vi "Main.vi"() -> ()   [LabVIEW 2011]
uses:
  Typedefs/Queue.ctl
  Typedefs/Queue cluster.ctl
  Typedefs/Cell details array.ctl
  Typedefs/Cell details cluster.ctl
  Typedefs/Scan settings.ctl
  Typedefs/StateEnum.ctl
panel:
  out "Server Status:":string
  out "Cell Settings Array 5":T1=[{"Measure?"=TRUE, "Area (cm^2)"=0.0, "Cell Label"="", "Cell Description"="", "Time between scans (s)"=0.0, "Cell Position"=1, "Scan settings in queue"=0, "Sample holder"=1.0, "User name"=""}, {"Measure?"=TRUE, "Area (cm^2)"=0.0, "Cell Label"="", "Cell Description"="", "Time between scans (s)"=0.0, "Cell Position"=2, "Scan settings in queue"=0, "Sample holder"=1.0, "User name"=""}, {"Measure?"=TRUE, "Area (cm^2)"=0.0, "Cell Label"="", "Cell Description"="", "Time between scans (s)"=0.0, "Cell Position"=3, "Scan settings in queue"=0, "Sample holder"=1.0, "User name"=""}, {"Measure?"=TRUE, "Area (cm^2)"=0.0, "Cell Label"="", "Cell Description"="", "Time between scans (s)"=0.0, "Cell Position"=4, "Scan settings in queue"=0, "Sample holder"=1.0, "User name"=""}, {"Measure?"=TRUE, "Area (cm^2)"=0.0, "Cell Label"="", "Cell Description"="", "Time between scans (s)"=0.0, "Cell Position"=5, "Scan settings in queue"=0, "Sample holder"=1.0, "User name"=""}, {"Measure?"=TRUE, "Area (cm^2)"=0.0, "Cell Label"="", "Cell Description"="", "Time between scans (s)"=0.0, "Cell Position"=6, "Scan settings in queue"=0, "Sample holder"=1.0, "User name"=""}, {"Measure?"=TRUE, "Area (cm^2)"=0.0, "Cell Label"="", "Cell Description"="", "Time between scans (s)"=0.0, "Cell Position"=7, "Scan settings in queue"=0, "Sample holder"=1.0, "User name"=""}, {"Measure?"=TRUE, "Area (cm^2)"=0.0, "Cell Label"="", "Cell Description"="", "Time between scans (s)"=0.0, "Cell Position"=8, "Scan settings in queue"=0, "Sample holder"=1.0, "User name"=""}, {"Measure?"=TRUE, "Area (cm^2)"=0.0, "Cell Label"="", "Cell Description"="", "Time between scans (s)"=0.0, "Cell Position"=9, "Scan settings in queue"=0, "Sample holder"=1.0, "User name"=""}, {"Measure?"=TRUE, "Area (cm^2)"=0.0, "Cell Label"="", "Cell Description"="", "Time between scans (s)"=0.0, "Cell Position"=10, "Scan settings in queue"=0, "Sample holder"=1.0, "User name"=""}, {"Measure?"=TRUE, "Area (cm^2)"=0.0, "Cell Label"="", "Cell Description"="", "Time between scans (s)"=0.0, "Cell Position"=11, "Scan settings in queue"=0, "Sample holder"=1.0, "User name"=""}, {"Measure?"=TRUE, "Area (cm^2)"=0.0, "Cell Label"="", "Cell Description"="", "Time between scans (s)"=0.0, "Cell Position"=12, "Scan settings in queue"=0, "Sample holder"=1.0, "User name"=""}, {"Measure?"=TRUE, "Area (cm^2)"=0.0, "Cell Label"="", "Cell Description"="", "Time between scans (s)"=0.0, "Cell Position"=13, "Scan settings in queue"=0, "Sample holder"=1.0, "User name"=""}, {"Measure?"=TRUE, "Area (cm^2)"=0.0, "Cell Label"="", "Cell Description"="", "Time between scans (s)"=0.0, "Cell Position"=14, "Scan settings in queue"=0, "Sample holder"=1.0, "User name"=""}, {"Measure?"=TRUE, "Area (cm^2)"=0.0, "Cell Label"="", "Cell Description"="", "Time between scans (s)"=0.0, "Cell Position"=15, "Scan settings in queue"=0, "Sample holder"=1.0, "User name"=""}, {"Measure?"=TRUE, "Area (cm^2)"=0.0, "Cell Label"="", "Cell Description"="", "Time between scans (s)"=0.0, "Cell Position"=16, "Scan settings in queue"=0, "Sample holder"=1.0, "User name"=""}] {"Scan settings in queue" items=["Standard"]}
  in  "Tab Control":T3(tab)
  in  "Cell Settings Array 1":T1=[{"Measure?"=TRUE, "Area (cm^2)"=0.0, "Cell Label"="", "Cell Description"="", "Time between scans (s)"=0.0, "Cell Position"=1, "Scan settings in queue"=0, "Sample holder"=1.0, "User name"=""}, {"Measure?"=TRUE, "Area (cm^2)"=0.0, "Cell Label"="", "Cell Description"="", "Time between scans (s)"=0.0, "Cell Position"=2, "Scan settings in queue"=0, "Sample holder"=1.0, "User name"=""}, {"Measure?"=TRUE, "Area (cm^2)"=0.0, "Cell Label"="", "Cell Description"="", "Time between scans (s)"=0.0, "Cell Position"=3, "Scan settings in queue"=0, "Sample holder"=1.0, "User name"=""}, {"Measure?"=TRUE, "Area (cm^2)"=0.0, "Cell Label"="", "Cell Description"="", "Time between scans (s)"=0.0, "Cell Position"=4, "Scan settings in queue"=0, "Sample holder"=1.0, "User name"=""}, {"Measure?"=TRUE, "Area (cm^2)"=0.0, "Cell Label"="", "Cell Description"="", "Time between scans (s)"=0.0, "Cell Position"=5, "Scan settings in queue"=0, "Sample holder"=1.0, "User name"=""}, {"Measure?"=TRUE, "Area (cm^2)"=0.0, "Cell Label"="", "Cell Description"="", "Time between scans (s)"=0.0, "Cell Position"=6, "Scan settings in queue"=0, "Sample holder"=1.0, "User name"=""}, {"Measure?"=TRUE, "Area (cm^2)"=0.0, "Cell Label"="", "Cell Description"="", "Time between scans (s)"=0.0, "Cell Position"=7, "Scan settings in queue"=0, "Sample holder"=1.0, "User name"=""}, {"Measure?"=TRUE, "Area (cm^2)"=0.0, "Cell Label"="", "Cell Description"="", "Time between scans (s)"=0.0, "Cell Position"=8, "Scan settings in queue"=0, "Sample holder"=1.0, "User name"=""}, {"Measure?"=TRUE, "Area (cm^2)"=0.0, "Cell Label"="", "Cell Description"="", "Time between scans (s)"=0.0, "Cell Position"=9, "Scan settings in queue"=0, "Sample holder"=1.0, "User name"=""}, {"Measure?"=TRUE, "Area (cm^2)"=0.0, "Cell Label"="", "Cell Description"="", "Time between scans (s)"=0.0, "Cell Position"=10, "Scan settings in queue"=0, "Sample holder"=1.0, "User name"=""}, {"Measure?"=TRUE, "Area (cm^2)"=0.0, "Cell Label"="", "Cell Description"="", "Time between scans (s)"=0.0, "Cell Position"=11, "Scan settings in queue"=0, "Sample holder"=1.0, "User name"=""}, {"Measure?"=TRUE, "Area (cm^2)"=0.0, "Cell Label"="", "Cell Description"="", "Time between scans (s)"=0.0, "Cell Position"=12, "Scan settings in queue"=0, "Sample holder"=1.0, "User name"=""}, {"Measure?"=TRUE, "Area (cm^2)"=0.0, "Cell Label"="", "Cell Description"="", "Time between scans (s)"=0.0, "Cell Position"=13, "Scan settings in queue"=0, "Sample holder"=1.0, "User name"=""}, {"Measure?"=TRUE, "Area (cm^2)"=0.0, "Cell Label"="", "Cell Description"="", "Time between scans (s)"=0.0, "Cell Position"=14, "Scan settings in queue"=0, "Sample holder"=1.0, "User name"=""}, {"Measure?"=TRUE, "Area (cm^2)"=0.0, "Cell Label"="", "Cell Description"="", "Time between scans (s)"=0.0, "Cell Position"=15, "Scan settings in queue"=0, "Sample holder"=1.0, "User name"=""}, {"Measure?"=TRUE, "Area (cm^2)"=0.0, "Cell Label"="", "Cell Description"="", "Time between scans (s)"=0.0, "Cell Position"=16, "Scan settings in queue"=0, "Sample holder"=1.0, "User name"=""}] {"Scan settings in queue" items=["David_Std", "Inverted", "Standard"]}
  in  "Upload from Spreadsheet?":bool
  in  "Upload Spreadsheet path":path=path "C:/Solar_Cell_Stability/Cell Details/Sample holder A.txt"
  in  "Save to Spreadsheet?":bool
  in  "Save Spreadsheet Path":path=path "C:/Solar_Cell_Stability/Cell Details/Sample holder A.txt"
  in  "Cell Settings Array 2":T1=[{"Measure?"=TRUE, "Area (cm^2)"=0.0, "Cell Label"="", "Cell Description"="", "Time between scans (s)"=0.0, "Cell Position"=1, "Scan settings in queue"=0, "Sample holder"=2.0, "User name"=""}, {"Measure?"=TRUE, "Area (cm^2)"=0.0, "Cell Label"="", "Cell Description"="", "Time between scans (s)"=0.0, "Cell Position"=2, "Scan settings in queue"=0, "Sample holder"=2.0, "User name"=""}, {"Measure?"=TRUE, "Area (cm^2)"=0.0, "Cell Label"="", "Cell Description"="", "Time between scans (s)"=0.0, "Cell Position"=3, "Scan settings in queue"=0, "Sample holder"=2.0, "User name"=""}, {"Measure?"=TRUE, "Area (cm^2)"=0.0, "Cell Label"="", "Cell Description"="", "Time between scans (s)"=0.0, "Cell Position"=4, "Scan settings in queue"=0, "Sample holder"=2.0, "User name"=""}, {"Measure?"=TRUE, "Area (cm^2)"=0.0, "Cell Label"="", "Cell Description"="", "Time between scans (s)"=0.0, "Cell Position"=5, "Scan settings in queue"=0, "Sample holder"=2.0, "User name"=""}, {"Measure?"=TRUE, "Area (cm^2)"=0.0, "Cell Label"="", "Cell Description"="", "Time between scans (s)"=0.0, "Cell Position"=6, "Scan settings in queue"=0, "Sample holder"=2.0, "User name"=""}, {"Measure?"=TRUE, "Area (cm^2)"=0.0, "Cell Label"="", "Cell Description"="", "Time between scans (s)"=0.0, "Cell Position"=7, "Scan settings in queue"=0, "Sample holder"=2.0, "User name"=""}, {"Measure?"=TRUE, "Area (cm^2)"=0.0, "Cell Label"="", "Cell Description"="", "Time between scans (s)"=0.0, "Cell Position"=8, "Scan settings in queue"=0, "Sample holder"=2.0, "User name"=""}, {"Measure?"=TRUE, "Area (cm^2)"=0.0, "Cell Label"="", "Cell Description"="", "Time between scans (s)"=0.0, "Cell Position"=9, "Scan settings in queue"=0, "Sample holder"=2.0, "User name"=""}, {"Measure?"=TRUE, "Area (cm^2)"=0.0, "Cell Label"="", "Cell Description"="", "Time between scans (s)"=0.0, "Cell Position"=10, "Scan settings in queue"=0, "Sample holder"=2.0, "User name"=""}, {"Measure?"=TRUE, "Area (cm^2)"=0.0, "Cell Label"="", "Cell Description"="", "Time between scans (s)"=0.0, "Cell Position"=11, "Scan settings in queue"=0, "Sample holder"=2.0, "User name"=""}, {"Measure?"=TRUE, "Area (cm^2)"=0.0, "Cell Label"="", "Cell Description"="", "Time between scans (s)"=0.0, "Cell Position"=12, "Scan settings in queue"=0, "Sample holder"=2.0, "User name"=""}, {"Measure?"=TRUE, "Area (cm^2)"=0.0, "Cell Label"="", "Cell Description"="", "Time between scans (s)"=0.0, "Cell Position"=13, "Scan settings in queue"=0, "Sample holder"=2.0, "User name"=""}, {"Measure?"=TRUE, "Area (cm^2)"=0.0, "Cell Label"="", "Cell Description"="", "Time between scans (s)"=0.0, "Cell Position"=14, "Scan settings in queue"=0, "Sample holder"=2.0, "User name"=""}, {"Measure?"=TRUE, "Area (cm^2)"=0.0, "Cell Label"="", "Cell Description"="", "Time between scans (s)"=0.0, "Cell Position"=15, "Scan settings in queue"=0, "Sample holder"=2.0, "User name"=""}, {"Measure?"=TRUE, "Area (cm^2)"=0.0, "Cell Label"="", "Cell Description"="", "Time between scans (s)"=0.0, "Cell Position"=16, "Scan settings in queue"=0, "Sample holder"=2.0, "User name"=""}] {"Scan settings in queue" items=["David_Std", "Inverted", "Standard"]}
  in  "Upload Spreadsheet path 2":path=path "C:/Solar_Cell_Stability/Cell Details/Sample holder B.txt"
  in  "Upload from Spreadsheet? 2":bool
  in  "Save Spreadsheet Path 2":path=path "C:/Solar_Cell_Stability/Cell Details/Sample holder B.txt"
  in  "Save to Spreadsheet?  2":bool
  in  "Cell Settings Array 3":T1=[{"Measure?"=TRUE, "Area (cm^2)"=0.0, "Cell Label"="", "Cell Description"="", "Time between scans (s)"=0.0, "Cell Position"=1, "Scan settings in queue"=0, "Sample holder"=3.0, "User name"=""}, {"Measure?"=TRUE, "Area (cm^2)"=0.0, "Cell Label"="", "Cell Description"="", "Time between scans (s)"=0.0, "Cell Position"=2, "Scan settings in queue"=0, "Sample holder"=3.0, "User name"=""}, {"Measure?"=TRUE, "Area (cm^2)"=0.0, "Cell Label"="", "Cell Description"="", "Time between scans (s)"=0.0, "Cell Position"=3, "Scan settings in queue"=0, "Sample holder"=3.0, "User name"=""}, {"Measure?"=TRUE, "Area (cm^2)"=0.0, "Cell Label"="", "Cell Description"="", "Time between scans (s)"=0.0, "Cell Position"=4, "Scan settings in queue"=0, "Sample holder"=3.0, "User name"=""}, {"Measure?"=TRUE, "Area (cm^2)"=0.0, "Cell Label"="", "Cell Description"="", "Time between scans (s)"=0.0, "Cell Position"=5, "Scan settings in queue"=0, "Sample holder"=3.0, "User name"=""}, {"Measure?"=TRUE, "Area (cm^2)"=0.0, "Cell Label"="", "Cell Description"="", "Time between scans (s)"=0.0, "Cell Position"=6, "Scan settings in queue"=0, "Sample holder"=3.0, "User name"=""}, {"Measure?"=TRUE, "Area (cm^2)"=0.0, "Cell Label"="", "Cell Description"="", "Time between scans (s)"=0.0, "Cell Position"=7, "Scan settings in queue"=0, "Sample holder"=3.0, "User name"=""}, {"Measure?"=TRUE, "Area (cm^2)"=0.0, "Cell Label"="", "Cell Description"="", "Time between scans (s)"=0.0, "Cell Position"=8, "Scan settings in queue"=0, "Sample holder"=3.0, "User name"=""}, {"Measure?"=TRUE, "Area (cm^2)"=0.0, "Cell Label"="", "Cell Description"="", "Time between scans (s)"=0.0, "Cell Position"=9, "Scan settings in queue"=0, "Sample holder"=3.0, "User name"=""}, {"Measure?"=TRUE, "Area (cm^2)"=0.0, "Cell Label"="", "Cell Description"="", "Time between scans (s)"=0.0, "Cell Position"=10, "Scan settings in queue"=0, "Sample holder"=3.0, "User name"=""}, {"Measure?"=TRUE, "Area (cm^2)"=0.0, "Cell Label"="", "Cell Description"="", "Time between scans (s)"=0.0, "Cell Position"=11, "Scan settings in queue"=0, "Sample holder"=3.0, "User name"=""}, {"Measure?"=TRUE, "Area (cm^2)"=0.0, "Cell Label"="", "Cell Description"="", "Time between scans (s)"=0.0, "Cell Position"=12, "Scan settings in queue"=0, "Sample holder"=3.0, "User name"=""}, {"Measure?"=TRUE, "Area (cm^2)"=0.0, "Cell Label"="", "Cell Description"="", "Time between scans (s)"=0.0, "Cell Position"=13, "Scan settings in queue"=0, "Sample holder"=3.0, "User name"=""}, {"Measure?"=TRUE, "Area (cm^2)"=0.0, "Cell Label"="", "Cell Description"="", "Time between scans (s)"=0.0, "Cell Position"=14, "Scan settings in queue"=0, "Sample holder"=3.0, "User name"=""}, {"Measure?"=TRUE, "Area (cm^2)"=0.0, "Cell Label"="", "Cell Description"="", "Time between scans (s)"=0.0, "Cell Position"=15, "Scan settings in queue"=0, "Sample holder"=3.0, "User name"=""}, {"Measure?"=TRUE, "Area (cm^2)"=0.0, "Cell Label"="", "Cell Description"="", "Time between scans (s)"=0.0, "Cell Position"=16, "Scan settings in queue"=0, "Sample holder"=3.0, "User name"=""}] {"Scan settings in queue" items=["David_Std", "Inverted", "Standard"]}
  in  "Upload Spreadsheet path 3":path=path "C:/Solar_Cell_Stability/Cell Details/Sample holder C.txt"
  in  "Upload from Spreadsheet? 3":bool
  in  "Save Spreadsheet Path 3":path=path "C:/Solar_Cell_Stability/Cell Details/Sample holder C.txt"
  in  "Save to Spreadsheet?  3":bool
  in  "Cell Settings Array 4":T1=[{"Measure?"=TRUE, "Area (cm^2)"=0.0, "Cell Label"="", "Cell Description"="", "Time between scans (s)"=0.0, "Cell Position"=1, "Scan settings in queue"=0, "Sample holder"=4.0, "User name"=""}, {"Measure?"=TRUE, "Area (cm^2)"=0.0, "Cell Label"="", "Cell Description"="", "Time between scans (s)"=0.0, "Cell Position"=2, "Scan settings in queue"=0, "Sample holder"=4.0, "User name"=""}, {"Measure?"=TRUE, "Area (cm^2)"=0.0, "Cell Label"="", "Cell Description"="", "Time between scans (s)"=0.0, "Cell Position"=3, "Scan settings in queue"=0, "Sample holder"=4.0, "User name"=""}, {"Measure?"=TRUE, "Area (cm^2)"=0.0, "Cell Label"="", "Cell Description"="", "Time between scans (s)"=0.0, "Cell Position"=4, "Scan settings in queue"=0, "Sample holder"=4.0, "User name"=""}, {"Measure?"=TRUE, "Area (cm^2)"=0.0, "Cell Label"="", "Cell Description"="", "Time between scans (s)"=0.0, "Cell Position"=5, "Scan settings in queue"=0, "Sample holder"=4.0, "User name"=""}, {"Measure?"=TRUE, "Area (cm^2)"=0.0, "Cell Label"="", "Cell Description"="", "Time between scans (s)"=0.0, "Cell Position"=6, "Scan settings in queue"=0, "Sample holder"=4.0, "User name"=""}, {"Measure?"=TRUE, "Area (cm^2)"=0.0, "Cell Label"="", "Cell Description"="", "Time between scans (s)"=0.0, "Cell Position"=7, "Scan settings in queue"=0, "Sample holder"=4.0, "User name"=""}, {"Measure?"=TRUE, "Area (cm^2)"=0.0, "Cell Label"="", "Cell Description"="", "Time between scans (s)"=0.0, "Cell Position"=8, "Scan settings in queue"=0, "Sample holder"=4.0, "User name"=""}, {"Measure?"=TRUE, "Area (cm^2)"=0.0, "Cell Label"="", "Cell Description"="", "Time between scans (s)"=0.0, "Cell Position"=9, "Scan settings in queue"=0, "Sample holder"=4.0, "User name"=""}, {"Measure?"=TRUE, "Area (cm^2)"=0.0, "Cell Label"="", "Cell Description"="", "Time between scans (s)"=0.0, "Cell Position"=10, "Scan settings in queue"=0, "Sample holder"=4.0, "User name"=""}, {"Measure?"=TRUE, "Area (cm^2)"=0.0, "Cell Label"="", "Cell Description"="", "Time between scans (s)"=0.0, "Cell Position"=11, "Scan settings in queue"=0, "Sample holder"=4.0, "User name"=""}, {"Measure?"=TRUE, "Area (cm^2)"=0.0, "Cell Label"="", "Cell Description"="", "Time between scans (s)"=0.0, "Cell Position"=12, "Scan settings in queue"=0, "Sample holder"=4.0, "User name"=""}, {"Measure?"=TRUE, "Area (cm^2)"=0.0, "Cell Label"="", "Cell Description"="", "Time between scans (s)"=0.0, "Cell Position"=13, "Scan settings in queue"=0, "Sample holder"=4.0, "User name"=""}, {"Measure?"=TRUE, "Area (cm^2)"=0.0, "Cell Label"="", "Cell Description"="", "Time between scans (s)"=0.0, "Cell Position"=14, "Scan settings in queue"=0, "Sample holder"=4.0, "User name"=""}, {"Measure?"=TRUE, "Area (cm^2)"=0.0, "Cell Label"="", "Cell Description"="", "Time between scans (s)"=0.0, "Cell Position"=15, "Scan settings in queue"=0, "Sample holder"=4.0, "User name"=""}, {"Measure?"=TRUE, "Area (cm^2)"=0.0, "Cell Label"="", "Cell Description"="", "Time between scans (s)"=0.0, "Cell Position"=16, "Scan settings in queue"=0, "Sample holder"=4.0, "User name"=""}] {"Scan settings in queue" items=["David_Std", "Inverted", "Standard"]}
  in  "Upload Spreadsheet path 4":path=path "C:/Solar_Cell_Stability/Cell Details/Sample holder D.txt"
  in  "Upload from Spreadsheet? 4":bool
  in  "Save Spreadsheet Path 4":path=path "C:/Solar_Cell_Stability/Cell Details/Sample holder D.txt"
  in  "Save to Spreadsheet?  4":bool
  in  "Stop Scan":bool
  in  "Start Scan":bool
  out "Table":string[][](table)
  in  "Upload to the Queue":bool
  in  "Stop Scan 2":bool
  out "J-V Curve":cluster{"Y":dbl[], "Y":dbl[]}[](graph)
  out "Max. Power Stabilization":cluster{"Y":dbl[], "Y":dbl[]}[](graph)
  in  "Scan Settings JV":T4={"Light intensity (Suns)"=1.0, "Pre-bias time (s)"=5.0, "Maximum voltage (V)"=0.0, "Minimum voltage (V)"=-1.4, "Range Options"=0, "1st scan FB to SC?"=TRUE, "Step Size (V)"=0.01, "Source Delay (s)"=0.01, "Inverted device"=FALSE, "Measure stabilized power output"=TRUE, "Stabilzation time (s)"=40.0, "Use Vmp from JV scan"=TRUE, "Stabization voltage (V)"=0.8, "Only stabilize best pixels"=TRUE, "Number of pixels to stabilize \nper substrate"=0, "Stabilization time step (s)"=1.0, "Use max power tracking"=FALSE, "Pre-bias voltage (V)"=-1.4, "No. of data point averages"=1.0, "No. of J-V averages"=1.0, "Integration time (ms)"=200.0} {"Integration time (ms)" min=0.2 max=200.0; "Number of pixels to stabilize \nper substrate" items=["1", "2", "3", "4", "5", "6", "7", "8"]; "Range Options" items=["Auto Range", "100 uA", "1 mA", "10 mA", "100 mA", "1A"]}
  in  "Save new settings as...":string
  in  "Save new settings":bool
  in  "Show saved settings":u16(ring) items=["David_Std", "Inverted", "Standard"]
  in  "Queue":T5 {"Scan settings in queue" items=["David_Std", "Inverted", "Standard"]; "Time of the last scan (s)" format="%<%H:%M:%S>t"; "When did you stick it in?" format="%<%H:%M:%S>t"; "Time to next scan (s)" format="%<%H:%M:%S>t"; "Time in rig (s)" format="%<%H:%M:%S>t"}
  out "TIMER":dbl format="%<%H:%M:%S>t"
  # "Cell Ageing"
  # "Time between Scans (s)"
  # "Area\n(cm^2)"
  # "Cell\nPosition"
  # "Sample\nHolder"
  # "On = working\nOff = not working"
  # "Label"
  # "User Name"
  # "Comment"
  # "Scan Settings"
  # "Time between Scans (s)"
  # "Area\n(cm^2)"
  # "Cell\nPosition"
  # "Sample\nHolder"
  # "On = working\nOff = not working"
  # "Label"
  # "User Name"
  # "Comment"
  # "Scan Settings"
  # "Time between Scans (s)"
  # "Area\n(cm^2)"
  # "Cell\nPosition"
  # "Sample\nHolder"
  # "On = working\nOff = not working"
  # "Label"
  # "User Name"
  # "Comment"
  # "Scan Settings"
  # "Time between Scans (s)"
  # "Area\n(cm^2)"
  # "Cell\nPosition"
  # "Sample\nHolder"
  # "On = working\nOff = not working"
  # "Label"
  # "User Name"
  # "Comment"
  # "Scan Settings"
  # "Time\n(s)"
  # "Light\nintensity"
  # "Cell\nLabel"
  # "Pixel\nNo."
  # "Scan\nNo."
  # "File\nPath"
  # "Area"
  # "Jsc"
  # "Voc"
  # "PCE"
  # "FF"
  # "Vmp"
  # "Comment"
  # "N.B. Voltage is applied to TCO electrode,\ni.e. the power generating quadrant is at \nnegative voltage for standard devices but \nat positive voltage for inverted devices."
  # "Area\n(cm^2)"
  # "Scan\nwait (s)"
  # "Cell \nposition"
  # "Time in rig\n(hrs)"
  # "Time to next scan (hrs)"
  # "Scan\nnumber"
  # "Time\nZero"
  # "Time of \nlast scan"
  # "Sample\nHolder"
  # "On = working\nOff = not working"
  # "Label"
  # "User"
  # "Comment"
  # "Scan Settings"
  # "WARNING: Deviating from these instructions may have serious consequences including massive data loss!\n\n\nBASIC OPERATION:\n\nFill out the cell details for each cell in each sample holder on the \"Sample Holder #\" tabs. For easy data analysis later, add an experiment indicator to\nthe \"Comments\" field. Be sure to complete all the information for each cell. If any boxes are blank, that cell won't be measured.\n\nGo to the \"Start/Stop Scan\" tab. Click the \"Initialise/Refresh Queue\" button. Check the \"Queue\" tab to make sure the the cell details have been added.\n\nOn the \"Start/Stop Scan\" tab click the \"Start Scan\" button. The cells in the queue will start to be measured.\n\n\n\nTO ADD CUSTOM SCAN SETTINGS:\n\nGo to the \"Scan Settings\" tab.\n\nInsert a new name into the \"Scan Setting Name\" box. Fill out the details in the pane and then press \"Save\". Your new settings are now accessible to\nselect when filling in the sample details in the \"Sample Holder #\" tabs.\n\nExisting settings can be viewed by selecting the appropriate option from the \"Show Scan Settings\" dropdown box.\n\n\n\nTO ADD/REMOVE/SWAP CELLS AND CONTINUE MEASUREMENT:\n\nGo to the \"Start/Stop Scan\" tab. Click the \"Stop Scan\" button. Wait for all the pixels on the current quad to finish measuring.\n\nAdd/change the required cells and repeat \"Basic Operation\".\n\n\n\nADDITIONAL INFORMATION\n\nDuring the measurement, only the \"Stop Scan\" button is functional. No changes can be made whilst measurements are running. Any attempts to \npress other buttons during measurements will result in a program crash.\n\nYou cannot update the comments box once a cell has been uploaded to the queue."
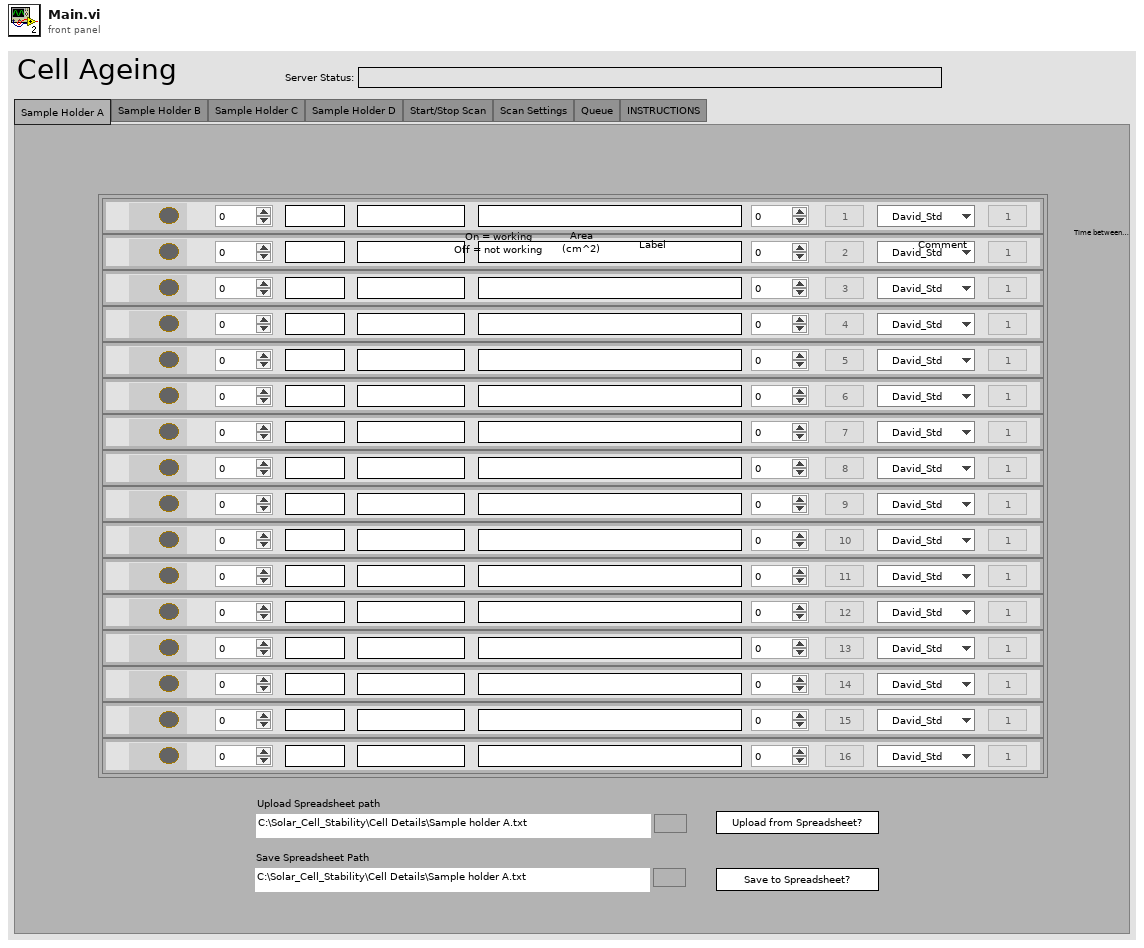
[diagram p1: front panel]
types:
  T1 = typedef "Cell details array.ctl" = T2[]
  T2 = typedef "Cell details cluster.ctl" = cluster{"Measure?":bool, "Area (cm^2)":dbl, "Cell Label":string, "Cell Description":string, "Time between scans (s)":dbl, "Cell Position":i32, "Scan settings in queue":u16, "Sample holder":dbl, "User name":string}
  T3 = enum32{"Sample Holder A", "Sample Holder B", "Sample Holder C", "Sample Holder D", "Start/Stop Scan", "Scan Settings", "Queue", "INSTRUCTIONS"}
  T4 = typedef "Scan settings.ctl" = cluster{"Light intensity (Suns)":dbl, "Pre-bias time (s)":dbl, "Maximum voltage (V)":dbl, "Minimum voltage (V)":dbl, "Range Options":u16, "1st scan FB to SC?":bool, "Step Size (V)":dbl, "Source Delay (s)":dbl, "Inverted device":bool, "Measure stabilized power output":bool, "Stabilzation time (s)":dbl, "Use Vmp from JV scan":bool, "Stabization voltage (V)":dbl, "Only stabilize best pixels":bool, "Number of pixels to stabilize \nper substrate":u16, "Stabilization time step (s)":dbl, "Use max power tracking":bool, "Pre-bias voltage (V)":dbl, "No. of data point averages":dbl, "No. of J-V averages":dbl, "Integration time (ms)":dbl}
  T5 = typedef "Queue.ctl" = T6[]
  T6 = typedef "Queue cluster.ctl" = cluster{"Measure?":bool, "Area (cm^2)":dbl, "Cell Label":string, "Cell Description":string, "Cell Position":i32, "Time in rig (s)":dbl, "Time to next scan (s)":dbl, "Scan number":dbl, "When did you stick it in?":dbl, "Time between scans (s)":dbl, "Time of the last scan (s)":dbl, "Scan settings in queue":u16, "Sample Holder":dbl, "User Name":string}
  T7 = typedef "StateEnum.ctl" = enum16{"Idle", "Measure"}
  T8 = enum8{"Enabled", "Disabled", "Disabled and Grayed Out"}
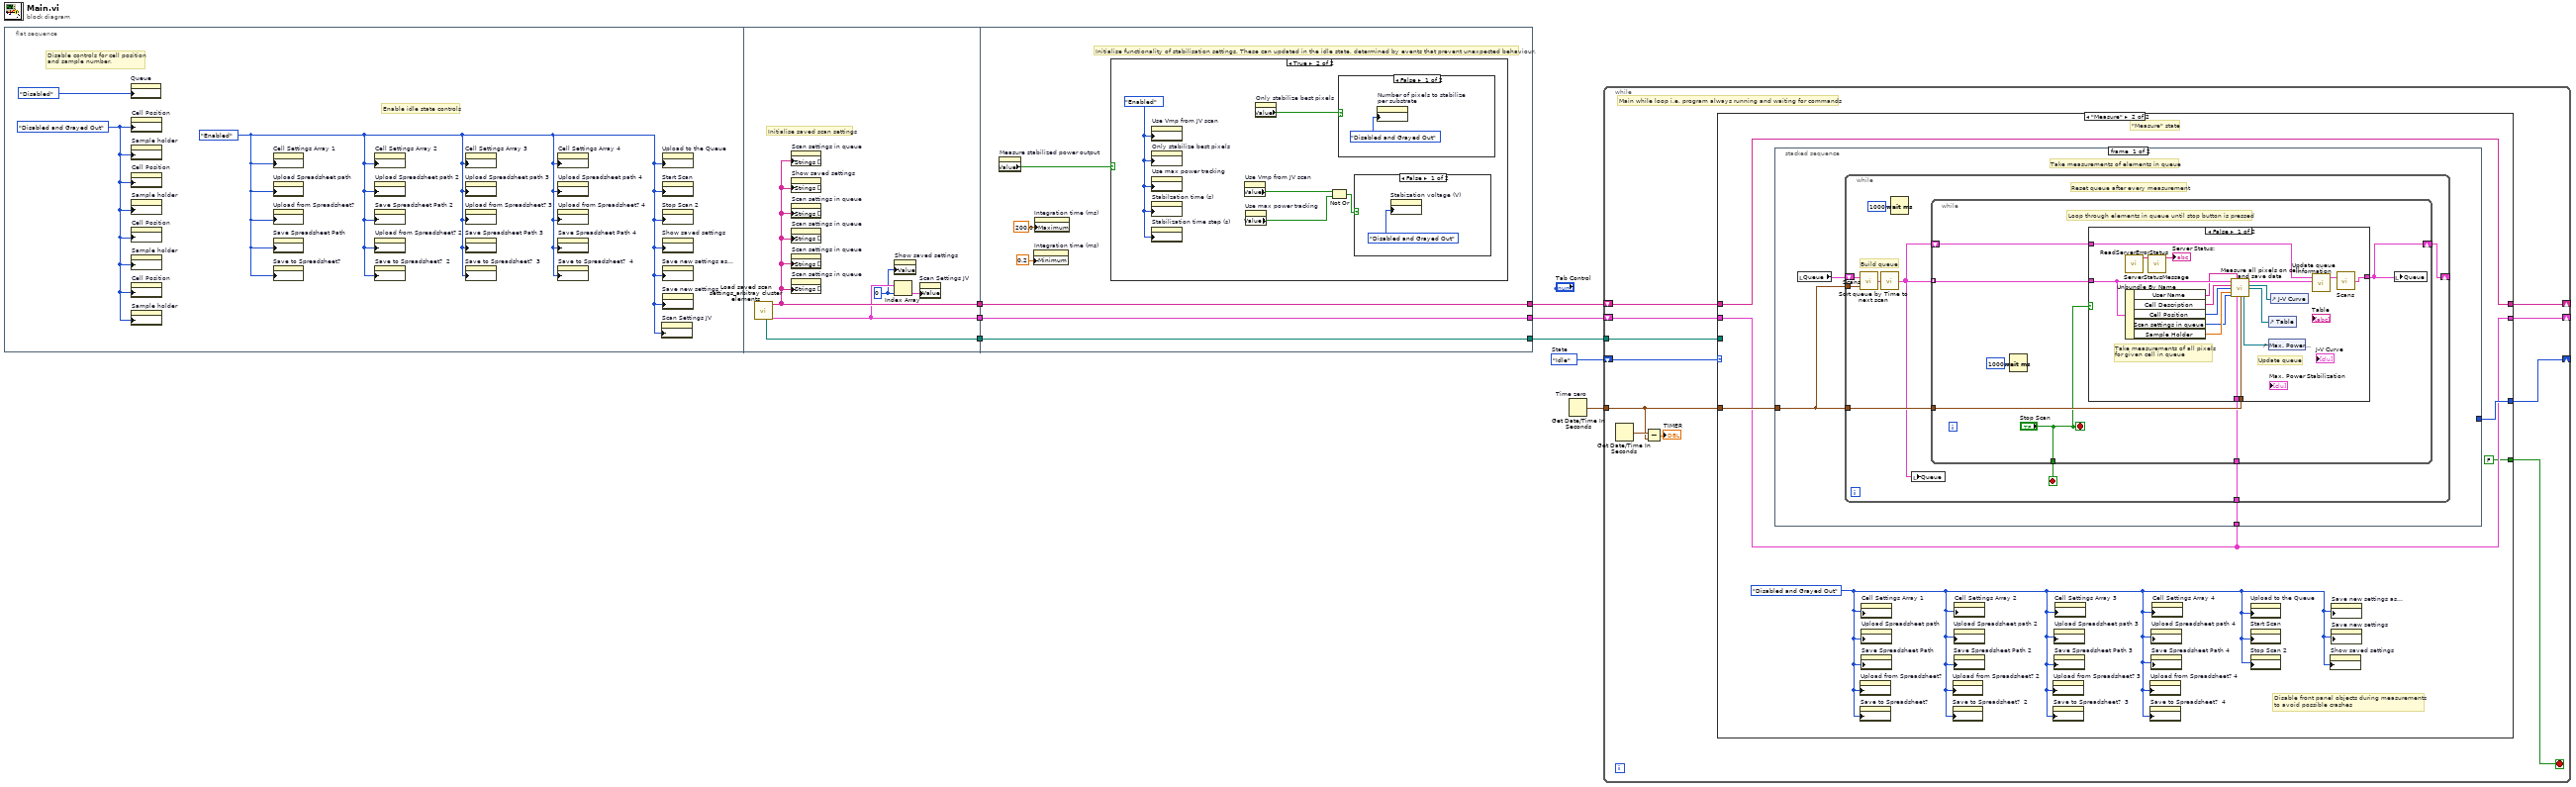
[diagram p0: block diagram]
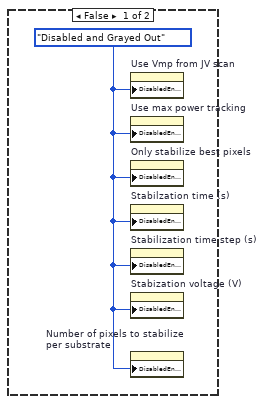
[diagram p2: hidden frame]
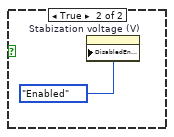
[diagram p3: hidden frame]
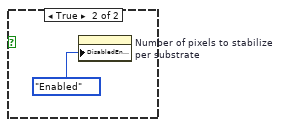
[diagram p4: hidden frame]
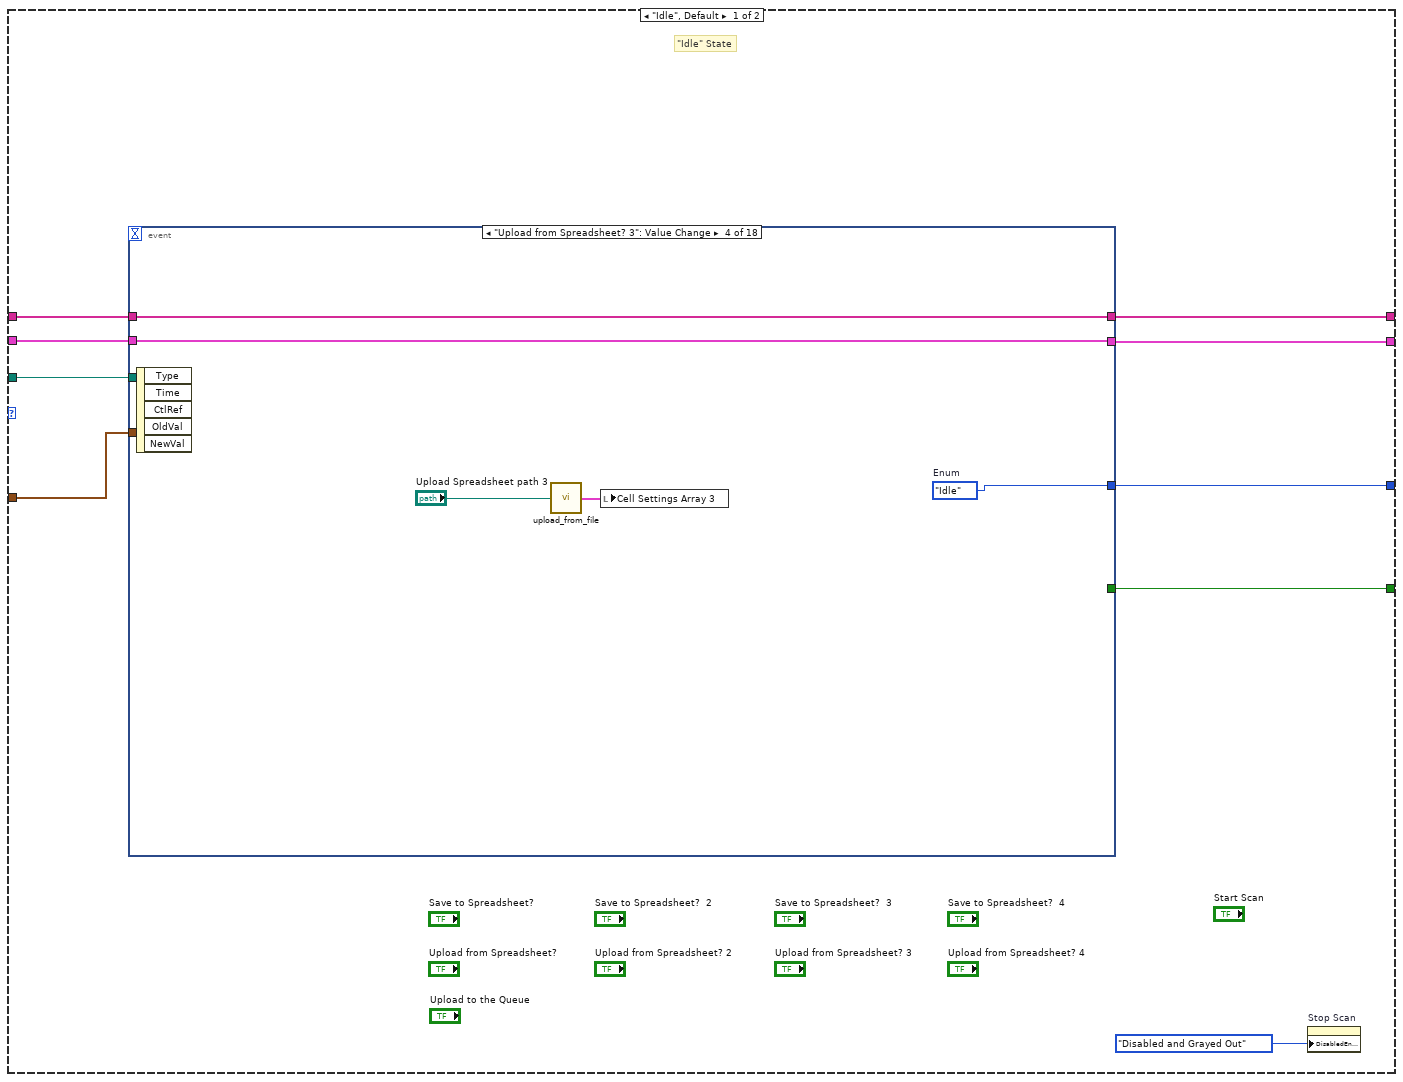
[diagram p5: hidden frame]
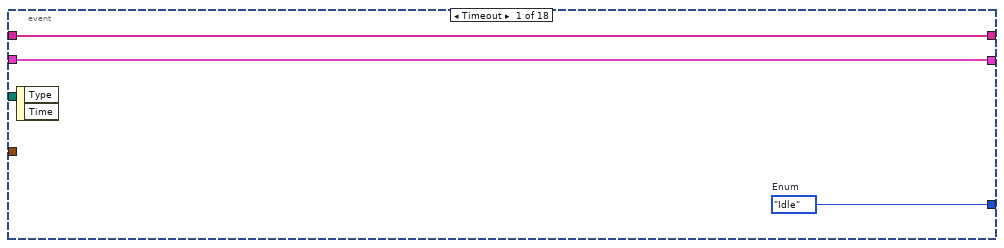
[diagram p6: hidden frame]
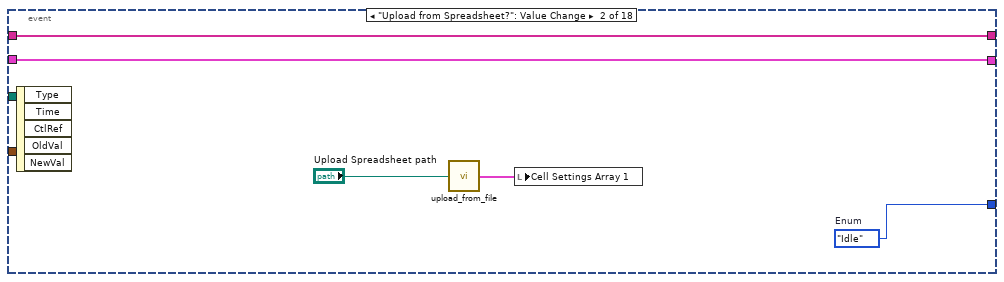
[diagram p7: hidden frame]
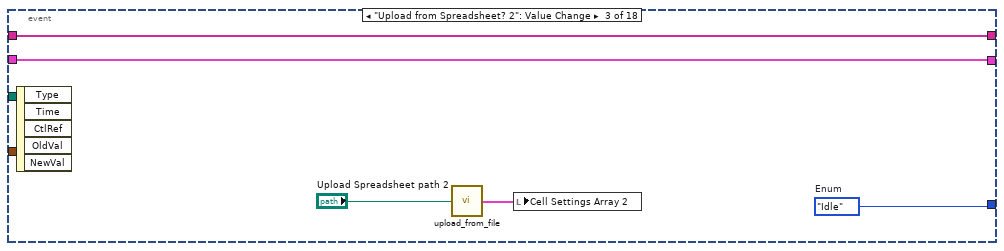
[diagram p8: hidden frame]
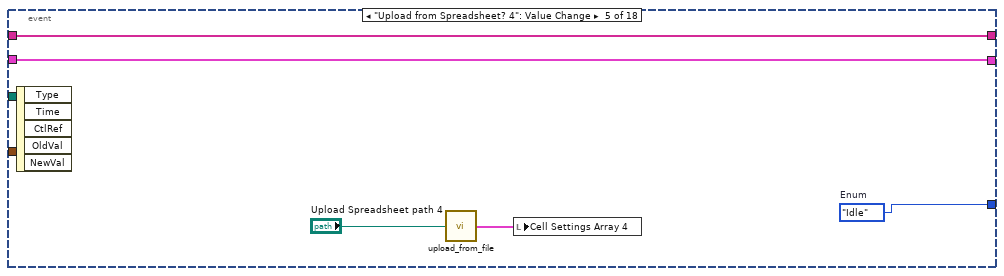
[diagram p9: hidden frame]
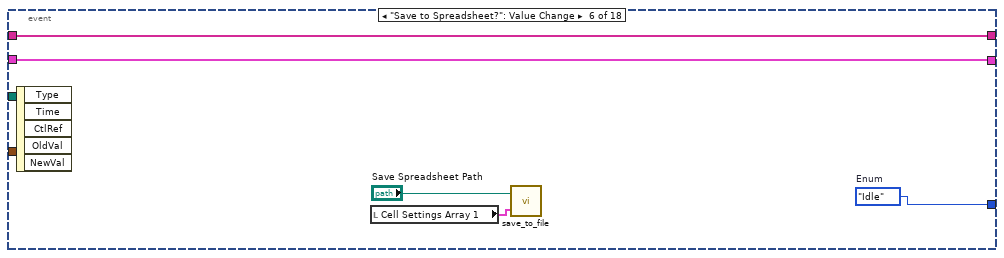
[diagram p10: hidden frame]
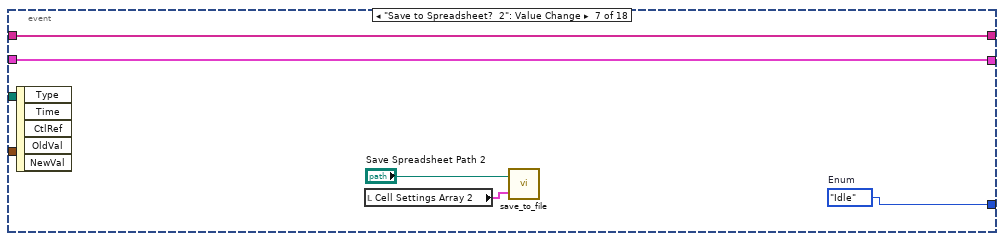
[diagram p11: hidden frame]
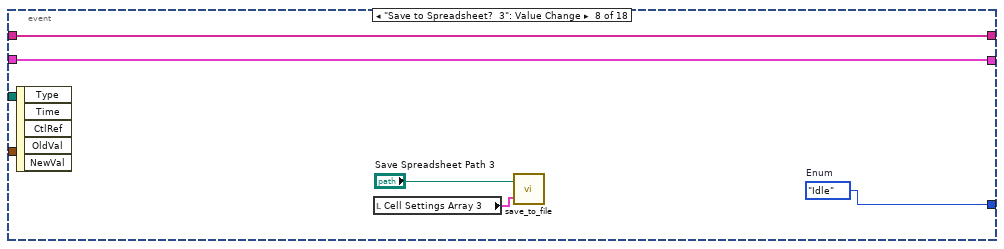
[diagram p12: hidden frame]
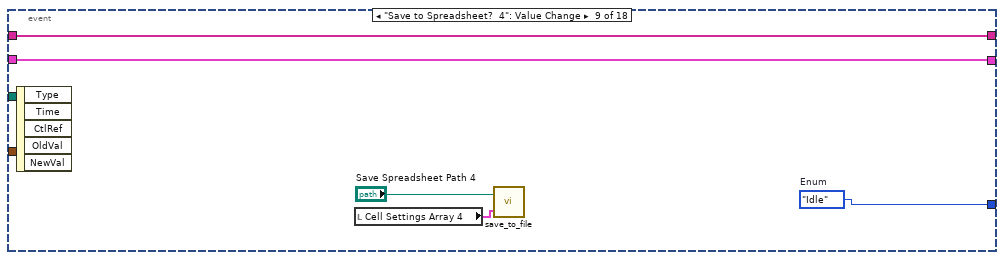
[diagram p13: hidden frame]
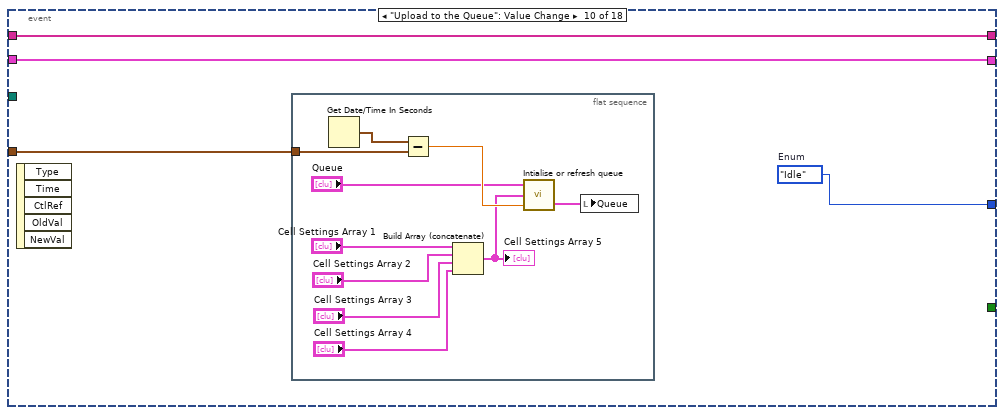
[diagram p14: hidden frame]
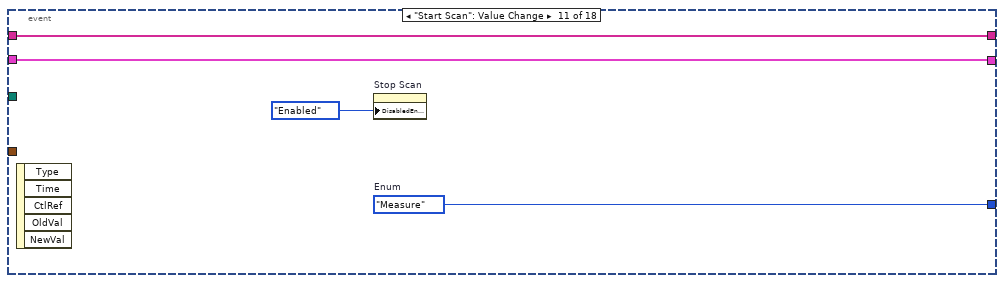
[diagram p15: hidden frame]
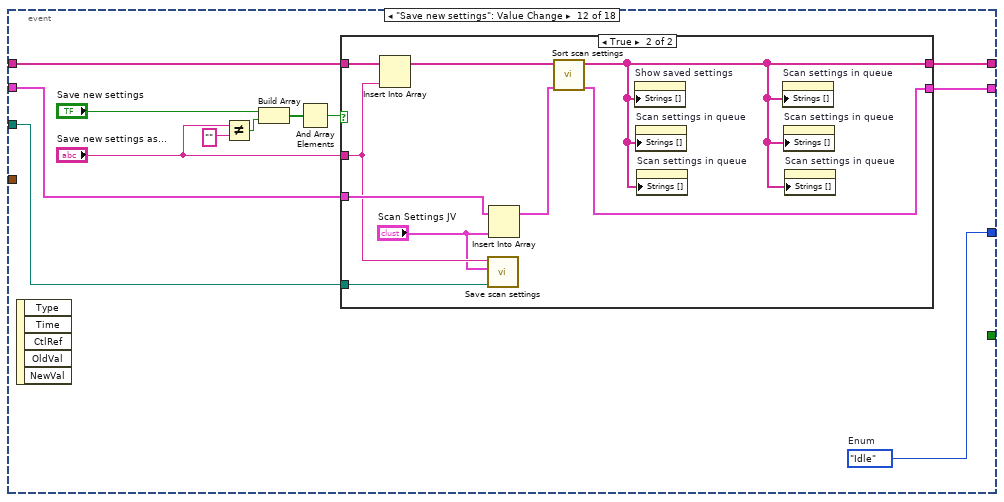
[diagram p16: hidden frame]
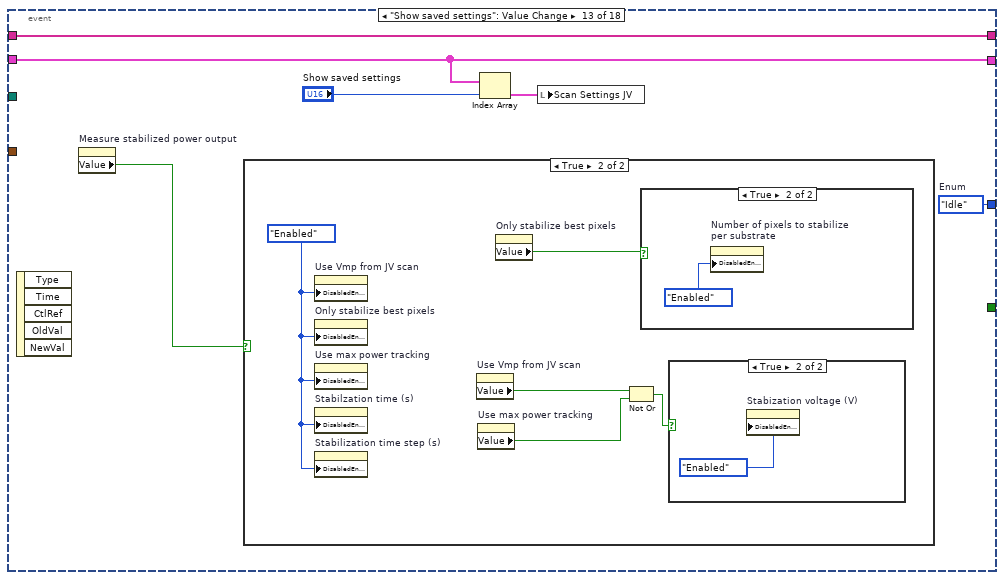
[diagram p18: hidden frame]
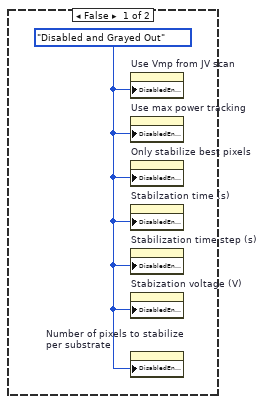
[diagram p19: hidden frame]
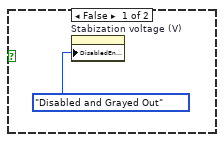
[diagram p20: hidden frame]
diagram:
  w7 = StateEnum."Idle"  # State
  n1 = flat-sequence {
    tunnel: [w16] -> w3
    tunnel: [w14] -> w2
    tunnel: [w15] -> w1
    tunnel: [w20] -> w4
    tunnel: [w21] -> w5
    tunnel: [w22] -> w6
    tunnel: w3 -> [w22]
    tunnel: w2 -> [w21]
    tunnel: w1 -> [w20]
    frame #0 {
      w10 = T8."Disabled and Grayed Out" ("Disabled")
      w11 = T8."Enabled" ("Disabled")
      # "Disable controls for cell position\nand sample number."
      # "Enable idle state controls"
      n2 = property on="Queue" class="Arr (strict)"("DisabledEnum"=T8."Disabled" ("Disabled")) -> ()  [unwired: 2 in, 2 out]
      n3 = property on="Cell Position" class="DigNum (strict)"("DisabledEnum"=w10) -> ()  [unwired: 2 in, 2 out]
      n4 = property on="Sample holder" class="DigNum (strict)"("DisabledEnum"=w10) -> ()  [unwired: 2 in, 2 out]
      n5 = property on="Cell Position" class="DigNum (strict)"("DisabledEnum"=w10) -> ()  [unwired: 2 in, 2 out]
      n6 = property on="Sample holder" class="DigNum (strict)"("DisabledEnum"=w10) -> ()  [unwired: 2 in, 2 out]
      n7 = property on="Cell Position" class="DigNum (strict)"("DisabledEnum"=w10) -> ()  [unwired: 2 in, 2 out]
      n8 = property on="Sample holder" class="DigNum (strict)"("DisabledEnum"=w10) -> ()  [unwired: 2 in, 2 out]
      n9 = property on="Cell Position" class="DigNum (strict)"("DisabledEnum"=w10) -> ()  [unwired: 2 in, 2 out]
      n10 = property on="Sample holder" class="DigNum (strict)"("DisabledEnum"=w10) -> ()  [unwired: 2 in, 2 out]
      n11 = property on="Cell Settings Array 1" class="Arr (strict)"("DisabledEnum"=w11) -> ()  [unwired: 2 in, 2 out]
      n12 = property on="Upload Spreadsheet path" class="Path"("DisabledEnum"=w11) -> ()  [unwired: 2 in, 2 out]
      n13 = property on="Upload from Spreadsheet?" class="Bool"("DisabledEnum"=w11) -> ()  [unwired: 2 in, 2 out]
      n14 = property on="Save Spreadsheet Path" class="Path"("DisabledEnum"=w11) -> ()  [unwired: 2 in, 2 out]
      n15 = property on="Save to Spreadsheet?" class="Bool"("DisabledEnum"=w11) -> ()  [unwired: 2 in, 2 out]
      n16 = property on="Cell Settings Array 2" class="Arr (strict)"("DisabledEnum"=w11) -> ()  [unwired: 2 in, 2 out]
      n17 = property on="Upload Spreadsheet path 2" class="Path"("DisabledEnum"=w11) -> ()  [unwired: 2 in, 2 out]
      n18 = property on="Save Spreadsheet Path 2" class="Path"("DisabledEnum"=w11) -> ()  [unwired: 2 in, 2 out]
      n19 = property on="Upload from Spreadsheet? 2" class="Bool"("DisabledEnum"=w11) -> ()  [unwired: 2 in, 2 out]
      n20 = property on="Save to Spreadsheet?  2" class="Bool"("DisabledEnum"=w11) -> ()  [unwired: 2 in, 2 out]
      n21 = property on="Cell Settings Array 3" class="Arr (strict)"("DisabledEnum"=w11) -> ()  [unwired: 2 in, 2 out]
      n22 = property on="Upload Spreadsheet path 3" class="Path"("DisabledEnum"=w11) -> ()  [unwired: 2 in, 2 out]
      n23 = property on="Upload from Spreadsheet? 3" class="Bool"("DisabledEnum"=w11) -> ()  [unwired: 2 in, 2 out]
      n24 = property on="Save Spreadsheet Path 3" class="Path"("DisabledEnum"=w11) -> ()  [unwired: 2 in, 2 out]
      n25 = property on="Save to Spreadsheet?  3" class="Bool"("DisabledEnum"=w11) -> ()  [unwired: 2 in, 2 out]
      n26 = property on="Cell Settings Array 4" class="Arr (strict)"("DisabledEnum"=w11) -> ()  [unwired: 2 in, 2 out]
      n27 = property on="Upload Spreadsheet path 4" class="Path"("DisabledEnum"=w11) -> ()  [unwired: 2 in, 2 out]
      n28 = property on="Upload from Spreadsheet? 4" class="Bool"("DisabledEnum"=w11) -> ()  [unwired: 2 in, 2 out]
      n29 = property on="Save Spreadsheet Path 4" class="Path"("DisabledEnum"=w11) -> ()  [unwired: 2 in, 2 out]
      n30 = property on="Save to Spreadsheet?  4" class="Bool"("DisabledEnum"=w11) -> ()  [unwired: 2 in, 2 out]
      n31 = property on="Scan Settings JV" class="Clust (strict)"("DisabledEnum"=w11) -> ()  [unwired: 2 in, 2 out]
      n32 = property on="Upload to the Queue" class="Bool (strict)"("DisabledEnum"=w11) -> ()  [unwired: 2 in, 2 out]
      n33 = property on="Start Scan" class="Bool"("DisabledEnum"=w11) -> ()  [unwired: 2 in, 2 out]
      n34 = property on="Stop Scan 2" class="Bool"("DisabledEnum"=w11) -> ()  [unwired: 2 in, 2 out]
      n35 = property on="Show saved settings" class="Ring (strict)"("DisabledEnum"=w11) -> ()  [unwired: 2 in, 2 out]
      n36 = property on="Save new settings as..." class="Str"("DisabledEnum"=w11) -> ()  [unwired: 2 in, 2 out]
      n37 = property on="Save new settings" class="Bool"("DisabledEnum"=w11) -> ()  [unwired: 2 in, 2 out]
    }
    frame #1 {
      w12 = 0 ("index")
      # "Initialise saved scan settings"
      n38 = call "Load saved scan settings_arbitray cluster elements.vi"() -> ("Scan settings array"=w14:T4[], "Scan settings name array"=w16:string[], "Settings folder path"=w15:path)  [unwired: 9 in]
      n39 = property on="Scan settings in queue" class="Ring (strict)"("Strings []"=w16) -> ()  [unwired: 2 in, 2 out]
      n40 = property on="Show saved settings" class="Ring (strict)"("Strings []"=w16) -> ()  [unwired: 2 in, 2 out]
      n41 = property on="Scan settings in queue" class="Ring (strict)"("Strings []"=w16) -> ()  [unwired: 2 in, 2 out]
      n42 = property on="Scan settings in queue" class="Ring (strict)"("Strings []"=w16) -> ()  [unwired: 2 in, 2 out]
      n43 = property on="Scan settings in queue" class="Ring (strict)"("Strings []"=w16) -> ()  [unwired: 2 in, 2 out]
      n44 = property on="Scan settings in queue" class="Ring (strict)"("Strings []"=w16) -> ()  [unwired: 2 in, 2 out]
      n45 = Index Array(array=w14, index=w12) -> (element=w13:T4)
      n46 = property on="Show saved settings" class="Ring (strict)"("Value"=w12) -> ()  [unwired: 2 in, 2 out]
      n47 = property on="Scan Settings JV" class="Clust (strict)"("Value"=w13) -> ()  [unwired: 2 in, 2 out]
    }
    frame #2 {
      # "Initialise functionality of stabilisation settings. These can updated in the idle state, determined by events that prevent unexpected behaviour."
      n48 = property on="Measure stabilized power output" class="Bool (strict)"() -> ("Value"=w19:bool)  [unwired: 2 in, 2 out]
      n49 = property on="Integration time (ms)" class="DigNum (strict)"("Minimum"=0.2 ("Data Entry Limits:Minimum")) -> ()  [unwired: 2 in, 2 out]
      n50 = property on="Integration time (ms)" class="DigNum (strict)"("Maximum"=200.0 ("Data Entry Limits:Maximum")) -> ()  [unwired: 2 in, 2 out]
      n51 = case shown="True" w19 {
        frame False {
          w23 = T8."Disabled and Grayed Out" ("Disabled")
          n52 = property on="Use Vmp from JV scan" class="Bool (strict)"("DisabledEnum"=w23) -> ()  [unwired: 2 in, 2 out]
          n53 = property on="Use max power tracking" class="Bool (strict)"("DisabledEnum"=w23) -> ()  [unwired: 2 in, 2 out]
          n54 = property on="Only stabilize best pixels" class="Bool (strict)"("DisabledEnum"=w23) -> ()  [unwired: 2 in, 2 out]
          n55 = property on="Stabilzation time (s)" class="DigNum (strict)"("DisabledEnum"=w23) -> ()  [unwired: 2 in, 2 out]
          n56 = property on="Stabilization time step (s)" class="DigNum (strict)"("DisabledEnum"=w23) -> ()  [unwired: 2 in, 2 out]
          n57 = property on="Stabization voltage (V)" class="DigNum (strict)"("DisabledEnum"=w23) -> ()  [unwired: 2 in, 2 out]
          n58 = property on="Number of pixels to stabilize \nper substrate" class="Ring (strict)"("DisabledEnum"=w23) -> ()  [unwired: 2 in, 2 out]
        }
        frame True {
          w28 = T8."Enabled" ("Disabled")
          n59 = property on="Use Vmp from JV scan" class="Bool (strict)"("DisabledEnum"=w28) -> ()  [unwired: 2 in, 2 out]
          n60 = property on="Only stabilize best pixels" class="Bool (strict)"("DisabledEnum"=w28) -> ()  [unwired: 2 in, 2 out]
          n61 = property on="Use max power tracking" class="Bool (strict)"("DisabledEnum"=w28) -> ()  [unwired: 2 in, 2 out]
          n62 = property on="Stabilzation time (s)" class="DigNum (strict)"("DisabledEnum"=w28) -> ()  [unwired: 2 in, 2 out]
          n63 = property on="Stabilization time step (s)" class="DigNum (strict)"("DisabledEnum"=w28) -> ()  [unwired: 2 in, 2 out]
          n64 = property on="Use Vmp from JV scan" class="Bool (strict)"() -> ("Value"=w26:bool)  [unwired: 2 in, 2 out]
          n65 = property on="Use max power tracking" class="Bool (strict)"() -> ("Value"=w25:bool)  [unwired: 2 in, 2 out]
          n66 = property on="Only stabilize best pixels" class="Bool (strict)"() -> ("Value"=w27:bool)  [unwired: 2 in, 2 out]
          n67 = Not Or(1:w25, 2:w26) -> (0:w24:bool)
          n68 = case shown="False" w27 {
            frame False {
              n69 = property on="Number of pixels to stabilize \nper substrate" class="Ring (strict)"("DisabledEnum"=T8."Disabled and Grayed Out" ("Disabled")) -> ()  [unwired: 2 in, 2 out]
            }
            frame True {
              n70 = property on="Number of pixels to stabilize \nper substrate" class="Ring (strict)"("DisabledEnum"=T8."Enabled" ("Disabled")) -> ()  [unwired: 2 in, 2 out]
            }
          }
          n71 = case shown="False" w24 {
            frame False {
              n72 = property on="Stabization voltage (V)" class="DigNum (strict)"("DisabledEnum"=T8."Disabled and Grayed Out" ("Disabled")) -> ()  [unwired: 2 in, 2 out]
            }
            frame True {
              n73 = property on="Stabization voltage (V)" class="DigNum (strict)"("DisabledEnum"=T8."Enabled" ("Disabled")) -> ()  [unwired: 2 in, 2 out]
            }
          }
        }
      }
    }
  }
  n74 = Get Date/Time In Seconds "Time zero"() -> (seconds since 1Jan1904=w8:timestamp)
  n75 = while {
    shift-right: [w37] -> _
    shift-left: w5 -> [w34]
    shift-right: [w38] -> _
    shift-left: w6 -> [w40]
    shift-right: [w41] -> _
    shift-left: w7 -> [w35]
    tunnel: w4 -> [w39]
    tunnel: w8 -> [w36]
    stop <- w33 stop-if-true
    # "Main while loop i.e. program always running and waiting for commands"
    n76 = Get Date/Time In Seconds() -> (seconds since 1Jan1904=w42:timestamp)
    n77 = Subtract(x=w42, y=w36) -> (x-y=→"TIMER":dbl)
    n78 = case shown="\"Measure\"" w35 {
      tunnel: [w51 w201] -> w41
      tunnel: w40 -> [w50 w199]
      tunnel: w34 -> [w45 w197]
      tunnel: w39 -> [w49 _]
      tunnel: [w48 w199] -> w38
      tunnel: [w47 w197] -> w37
      tunnel: w36 -> [w46 w200]
      tunnel: [w44 FALSE ("Stop Scan 2")] -> w33
      frame "Idle", Default {
        # "\"Idle\" State"
        n79 = event shown="[3] \"Upload from Spreadsheet? 3\": Value Change" {
          selector: _ -> [_ _ _ _ _ _ _ _ _ _ _ _ _ _ _ _ _ _]
          dyn-events: _ -> [_ _ _ _ _ _ _ _ _ _ _ _ _ _ _ _ _ _]
          timeout: _ -> [_ _ _ _ _ _ _ _ _ _ _ _ _ _ _ _ _ _]
          tunnel: [w55 w58 w63 w68 w73 w78 w83 w88 w93 w99 w113 w114 w139 _ _ _ _ _] -> w51
          tunnel: w50 -> [w54 w57 w62 w67 w72 w77 w82 w87 w92 w97 w112 w119 w142 w155 w173 w178 w187 _]
          tunnel: w45 -> [w53 w56 w61 w66 w71 w76 w81 w86 w91 w96 w111 w118 w141 w153 w172 w177 w186 _]
          tunnel: w49 -> [_ _ _ _ _ _ _ _ _ _ _ w117 _ _ _ _ _ _]
          tunnel: [w54 w57 w62 w67 w72 w77 w82 w87 w92 w97 w112 w116 w142 w156 w173 w178 w187 _] -> w48
          tunnel: [w53 w56 w61 w66 w71 w76 w81 w86 w91 w96 w111 w115 w141 w154 w172 w177 w186 _] -> w47
          tunnel: w46 -> [_ _ _ _ _ _ _ _ _ w98 _ _ _ _ _ _ _ _]
          tunnel: [_ _ _ _ _ _ _ _ _ _ _ _ _ _ _ _ _ "Stop Scan 2"] -> w44
          event Timeout {
            w55 = StateEnum."Idle"  # Enum
            n80 = event-data() -> ()  [unwired: 1 in, 2 out]
          }
          event "Upload from Spreadsheet?": Value Change {
            w58 = StateEnum."Idle"  # Enum
            n81 = event-data() -> ()  [unwired: 1 in, 5 out]
            n82 = call "upload_from_file.vi"("Spreadsheet path"="Upload Spreadsheet path") -> ("Cell Settings Array 4"=w59:T1)
            n83 = local write "Cell Settings Array 1"(w59) -> ()
          }
          event "Upload from Spreadsheet? 2": Value Change {
            w63 = StateEnum."Idle"  # Enum
            n84 = event-data() -> ()  [unwired: 1 in, 5 out]
            n85 = call "upload_from_file.vi"("Spreadsheet path"="Upload Spreadsheet path 2") -> ("Cell Settings Array 4"=w65:T1)
            n86 = local write "Cell Settings Array 2"(w65) -> ()
          }
          event "Upload from Spreadsheet? 3": Value Change {
            w68 = StateEnum."Idle"  # Enum
            n87 = event-data() -> ()  [unwired: 1 in, 5 out]
            n88 = call "upload_from_file.vi"("Spreadsheet path"="Upload Spreadsheet path 3") -> ("Cell Settings Array 4"=w70:T1)
            n89 = local write "Cell Settings Array 3"(w70) -> ()
          }
          event "Upload from Spreadsheet? 4": Value Change {
            w73 = StateEnum."Idle"  # Enum
            n90 = event-data() -> ()  [unwired: 1 in, 5 out]
            n91 = call "upload_from_file.vi"("Spreadsheet path"="Upload Spreadsheet path 4") -> ("Cell Settings Array 4"=w75:T1)
            n92 = local write "Cell Settings Array 4"(w75) -> ()
          }
          event "Save to Spreadsheet?": Value Change {
            w78 = StateEnum."Idle"  # Enum
            n93 = event-data() -> ()  [unwired: 1 in, 5 out]
            n94 = local read "Cell Settings Array 1"() -> (w80:T1)
            n95 = call "save_to_file.vi"("Cell Settings Array 4"=w80, "Save Path"="Save Spreadsheet Path") -> ()  [unwired: 1 in]
          }
          event "Save to Spreadsheet?  2": Value Change {
            w83 = StateEnum."Idle"  # Enum
            n96 = event-data() -> ()  [unwired: 1 in, 5 out]
            n97 = local read "Cell Settings Array 2"() -> (w85:T1)
            n98 = call "save_to_file.vi"("Cell Settings Array 4"=w85, "Save Path"="Save Spreadsheet Path 2") -> ()  [unwired: 1 in]
          }
          event "Save to Spreadsheet?  3": Value Change {
            w88 = StateEnum."Idle"  # Enum
            n99 = event-data() -> ()  [unwired: 1 in, 5 out]
            n100 = local read "Cell Settings Array 3"() -> (w89:T1)
            n101 = call "save_to_file.vi"("Cell Settings Array 4"=w89, "Save Path"="Save Spreadsheet Path 3") -> ()  [unwired: 1 in]
          }
          event "Save to Spreadsheet?  4": Value Change {
            w93 = StateEnum."Idle"  # Enum
            n102 = event-data() -> ()  [unwired: 1 in, 5 out]
            n103 = local read "Cell Settings Array 4"() -> (w94:T1)
            n104 = call "save_to_file.vi"("Cell Settings Array 4"=w94, "Save Path"="Save Spreadsheet Path 4") -> ()  [unwired: 1 in]
          }
          event "Upload to the Queue": Value Change {
            w99 = StateEnum."Idle"  # Enum
            n105 = event-data() -> ()  [unwired: 1 in, 5 out]
            n106 = flat-sequence {
              tunnel: w98 -> [w104]
              frame #0 {
                n107 = Get Date/Time In Seconds() -> (seconds since 1Jan1904=w109:timestamp)
                n108 = Subtract(x=w109, y=w104) -> (x-y=w108:dbl)
                n109 = Build Array (concatenate)("Cell Settings Array 1", "Cell Settings Array 2", "Cell Settings Array 3", "Cell Settings Array 4") -> (w100:T1)
                "Cell Settings Array 5" <- w100
                n110 = call "Intialise or refresh queue.vi"("When did you stick it in?"=w108, "Cell Settings Array"=w100, "Queue in"="Queue") -> ("Queue out"=w105:T5)  [unwired: 1 in]
                n111 = local write "Queue"(w105) -> ()
              }
            }
          }
          event "Start Scan": Value Change {
            w113 = StateEnum."Measure"  # Enum
            n112 = event-data() -> ()  [unwired: 1 in, 5 out]
            n113 = property on="Stop Scan" class="Bool"("DisabledEnum"=T8."Enabled" ("Disabled")) -> ()  [unwired: 2 in, 2 out]
          }
          event "Save new settings": Value Change {
            w114 = StateEnum."Idle"  # Enum
            n114 = event-data() -> ()  [unwired: 1 in, 5 out]
            n115 = Not Equal?(x="Save new settings as...", y="") -> (x != y?=w123:bool)
            n116 = Build Array("Save new settings", w123) -> (w124:bool[])
            n117 = And Array Elements(Boolean array=w124) -> (logical AND=w120:bool)
            n118 = case shown="True" w120 {
              tunnel: "Save new settings as..." -> [_ w134]
              tunnel: w119 -> [w127 w136]
              tunnel: w118 -> [w126 w135]
              tunnel: w117 -> [_ w133]
              tunnel: [w127 w130] -> w116
              tunnel: [w126 w128] -> w115
              frame False {
              }
              frame True {
                n119 = Insert Into Array(array=w136, new element=w134) -> (w131:string[])  [unwired: 1 in]
                n120 = call "Save scan settings.vi"("Path"=w133, "New scan settings"="Scan Settings JV", "New name"=w134) -> ()  [unwired: 9 in]
                n121 = Insert Into Array(array=w135, new element="Scan Settings JV") -> (w129:T4[])  [unwired: 1 in]
                n122 = call "Sort scan settings.vi"("Scan settings array"=w129, "Setting name array"=w131) -> ("Sorted settings array"=w128:T4[], "Sorted name array"=w130:string[])  [unwired: 7 in]
                n123 = property on="Show saved settings" class="Ring (strict)"("Strings []"=w130) -> ()  [unwired: 2 in, 2 out]
                n124 = property on="Scan settings in queue" class="Ring (strict)"("Strings []"=w130) -> ()  [unwired: 2 in, 2 out]
                n125 = property on="Scan settings in queue" class="Ring (strict)"("Strings []"=w130) -> ()  [unwired: 2 in, 2 out]
                n126 = property on="Scan settings in queue" class="Ring (strict)"("Strings []"=w130) -> ()  [unwired: 2 in, 2 out]
                n127 = property on="Scan settings in queue" class="Ring (strict)"("Strings []"=w130) -> ()  [unwired: 2 in, 2 out]
                n128 = property on="Scan settings in queue" class="Ring (strict)"("Strings []"=w130) -> ()  [unwired: 2 in, 2 out]
              }
            }
          }
          event "Show saved settings": Value Change {
            w139 = StateEnum."Idle"  # Enum
            n129 = event-data() -> ()  [unwired: 1 in, 5 out]
            n130 = property on="Measure stabilized power output" class="Bool (strict)"() -> ("Value"=w137:bool)  [unwired: 2 in, 2 out]
            n131 = case shown="True" w137 {
              frame False {
                w143 = T8."Disabled and Grayed Out" ("Disabled")
                n132 = property on="Use Vmp from JV scan" class="Bool (strict)"("DisabledEnum"=w143) -> ()  [unwired: 2 in, 2 out]
                n133 = property on="Use max power tracking" class="Bool (strict)"("DisabledEnum"=w143) -> ()  [unwired: 2 in, 2 out]
                n134 = property on="Only stabilize best pixels" class="Bool (strict)"("DisabledEnum"=w143) -> ()  [unwired: 2 in, 2 out]
                n135 = property on="Stabilzation time (s)" class="DigNum (strict)"("DisabledEnum"=w143) -> ()  [unwired: 2 in, 2 out]
                n136 = property on="Stabilization time step (s)" class="DigNum (strict)"("DisabledEnum"=w143) -> ()  [unwired: 2 in, 2 out]
                n137 = property on="Stabization voltage (V)" class="DigNum (strict)"("DisabledEnum"=w143) -> ()  [unwired: 2 in, 2 out]
                n138 = property on="Number of pixels to stabilize \nper substrate" class="Ring (strict)"("DisabledEnum"=w143) -> ()  [unwired: 2 in, 2 out]
              }
              frame True {
                w148 = T8."Enabled" ("Disabled")
                n139 = property on="Use Vmp from JV scan" class="Bool (strict)"("DisabledEnum"=w148) -> ()  [unwired: 2 in, 2 out]
                n140 = property on="Only stabilize best pixels" class="Bool (strict)"("DisabledEnum"=w148) -> ()  [unwired: 2 in, 2 out]
                n141 = property on="Use max power tracking" class="Bool (strict)"("DisabledEnum"=w148) -> ()  [unwired: 2 in, 2 out]
                n142 = property on="Stabilzation time (s)" class="DigNum (strict)"("DisabledEnum"=w148) -> ()  [unwired: 2 in, 2 out]
                n143 = property on="Stabilization time step (s)" class="DigNum (strict)"("DisabledEnum"=w148) -> ()  [unwired: 2 in, 2 out]
                n144 = property on="Use Vmp from JV scan" class="Bool (strict)"() -> ("Value"=w146:bool)  [unwired: 2 in, 2 out]
                n145 = property on="Use max power tracking" class="Bool (strict)"() -> ("Value"=w145:bool)  [unwired: 2 in, 2 out]
                n146 = property on="Only stabilize best pixels" class="Bool (strict)"() -> ("Value"=w147:bool)  [unwired: 2 in, 2 out]
                n147 = Not Or(1:w145, 2:w146) -> (0:w144:bool)
                n148 = case shown="True" w147 {
                  frame False {
                    n149 = property on="Number of pixels to stabilize \nper substrate" class="Ring (strict)"("DisabledEnum"=T8."Disabled and Grayed Out" ("Disabled")) -> ()  [unwired: 2 in, 2 out]
                  }
                  frame True {
                    n150 = property on="Number of pixels to stabilize \nper substrate" class="Ring (strict)"("DisabledEnum"=T8."Enabled" ("Disabled")) -> ()  [unwired: 2 in, 2 out]
                  }
                }
                n151 = case shown="True" w144 {
                  frame False {
                    n152 = property on="Stabization voltage (V)" class="DigNum (strict)"("DisabledEnum"=T8."Disabled and Grayed Out" ("Disabled")) -> ()  [unwired: 2 in, 2 out]
                  }
                  frame True {
                    n153 = property on="Stabization voltage (V)" class="DigNum (strict)"("DisabledEnum"=T8."Enabled" ("Disabled")) -> ()  [unwired: 2 in, 2 out]
                  }
                }
              }
            }
            n154 = Index Array(array=w141, index="Show saved settings") -> (element=w138:T4)
            n155 = local write "Scan Settings JV"(w138) -> ()
          }
          event Value Change {
            n156 = event-data() -> ()  [unwired: 1 in, 5 out]
            n157 = property on="Measure stabilized power output" class="Bool (strict)"() -> ("Value"=w157:bool)  [unwired: 2 in, 2 out]
            n158 = case shown="False" w157 {
              tunnel: [w159 w162] -> w156
              tunnel: w155 -> [w159 w162]
              tunnel: [w158 w161] -> w154
              tunnel: w153 -> [w158 w161]
              frame False {
                w160 = T8."Disabled and Grayed Out" ("Disabled")
                n159 = property on="Use Vmp from JV scan" class="Bool (strict)"("DisabledEnum"=w160) -> ()  [unwired: 2 in, 2 out]
                n160 = property on="Use max power tracking" class="Bool (strict)"("DisabledEnum"=w160) -> ()  [unwired: 2 in, 2 out]
                n161 = property on="Only stabilize best pixels" class="Bool (strict)"("DisabledEnum"=w160) -> ()  [unwired: 2 in, 2 out]
                n162 = property on="Stabilzation time (s)" class="DigNum (strict)"("DisabledEnum"=w160) -> ()  [unwired: 2 in, 2 out]
                n163 = property on="Stabilization time step (s)" class="DigNum (strict)"("DisabledEnum"=w160) -> ()  [unwired: 2 in, 2 out]
                n164 = property on="Stabization voltage (V)" class="DigNum (strict)"("DisabledEnum"=w160) -> ()  [unwired: 2 in, 2 out]
                n165 = property on="Number of pixels to stabilize \nper substrate" class="Ring (strict)"("DisabledEnum"=w160) -> ()  [unwired: 2 in, 2 out]
              }
              frame True {
                w167 = T8."Enabled" ("Disabled")
                n166 = property on="Only stabilize best pixels" class="Bool (strict)"("DisabledEnum"=w167) -> ()  [unwired: 2 in, 2 out]
                n167 = property on="Stabilzation time (s)" class="DigNum (strict)"("DisabledEnum"=w167) -> ()  [unwired: 2 in, 2 out]
                n168 = property on="Stabilization time step (s)" class="DigNum (strict)"("DisabledEnum"=w167) -> ()  [unwired: 2 in, 2 out]
                n169 = property on="Use Vmp from JV scan" class="Bool (strict)"("DisabledEnum"=w167) -> ()  [unwired: 2 in, 2 out]
                n170 = property on="Use max power tracking" class="Bool (strict)"("DisabledEnum"=w167) -> ()  [unwired: 2 in, 2 out]
                n171 = property on="Use max power tracking" class="Bool (strict)"() -> ("Value"=w164:bool)  [unwired: 2 in, 2 out]
                n172 = property on="Use Vmp from JV scan" class="Bool (strict)"() -> ("Value"=w165:bool)  [unwired: 2 in, 2 out]
                n173 = property on="Only stabilize best pixels" class="Bool (strict)"() -> ("Value"=w166:bool)  [unwired: 2 in, 2 out]
                n174 = Not Or(1:w164, 2:w165) -> (0:w163:bool)
                n175 = case shown="False" w166 {
                  frame False {
                    n176 = property on="Number of pixels to stabilize \nper substrate" class="Ring (strict)"("DisabledEnum"=T8."Disabled and Grayed Out" ("Disabled")) -> ()  [unwired: 2 in, 2 out]
                  }
                  frame True {
                    n177 = property on="Number of pixels to stabilize \nper substrate" class="Ring (strict)"("DisabledEnum"=T8."Enabled" ("Disabled")) -> ()  [unwired: 2 in, 2 out]
                  }
                }
                n178 = case shown="False" w163 {
                  frame False {
                    n179 = property on="Stabization voltage (V)" class="DigNum (strict)"("DisabledEnum"=T8."Disabled and Grayed Out" ("Disabled")) -> ()  [unwired: 2 in, 2 out]
                  }
                  frame True {
                    n180 = property on="Stabization voltage (V)" class="DigNum (strict)"("DisabledEnum"=T8."Enabled" ("Disabled")) -> ()  [unwired: 2 in, 2 out]
                  }
                }
              }
            }
          }
          event Value Change {
            n181 = event-data() -> ()  [unwired: 1 in, 5 out]
            n182 = property on="Only stabilize best pixels" class="Bool (strict)"() -> ("Value"=w174:bool)  [unwired: 2 in, 2 out]
            n183 = case shown="False" w174 {
              frame False {
                n184 = property on="Number of pixels to stabilize \nper substrate" class="Ring (strict)"("DisabledEnum"=T8."Disabled and Grayed Out" ("Disabled")) -> ()  [unwired: 2 in, 2 out]
              }
              frame True {
                n185 = property on="Number of pixels to stabilize \nper substrate" class="Ring (strict)"("DisabledEnum"=T8."Enabled" ("Disabled")) -> ()  [unwired: 2 in, 2 out]
              }
            }
          }
          event Value Change {
            n186 = event-data() -> ()  [unwired: 1 in, 5 out]
            n187 = property on="Use Vmp from JV scan" class="Bool (strict)"() -> ("Value"=w182:bool)  [unwired: 2 in, 2 out]
            n188 = case shown="True" w182 {
              frame False {
              }
              frame True {
                n189 = property on="Use max power tracking" class="Bool (strict)"("Value"=FALSE) -> ()  [unwired: 2 in, 2 out]
              }
            }
            n190 = property on="Use max power tracking" class="Bool (strict)"() -> ("Value"=w180:bool)  [unwired: 2 in, 2 out]
            n191 = property on="Use Vmp from JV scan" class="Bool (strict)"() -> ("Value"=w181:bool)  [unwired: 2 in, 2 out]
            n192 = Not Or(1:w180, 2:w181) -> (0:w179:bool)
            n193 = case shown="False" w179 {
              frame False {
                n194 = property on="Stabization voltage (V)" class="DigNum (strict)"("DisabledEnum"=T8."Disabled and Grayed Out" ("Disabled")) -> ()  [unwired: 2 in, 2 out]
              }
              frame True {
                n195 = property on="Stabization voltage (V)" class="DigNum (strict)"("DisabledEnum"=T8."Enabled" ("Disabled")) -> ()  [unwired: 2 in, 2 out]
              }
            }
          }
          event Value Change {
            n196 = event-data() -> ()  [unwired: 1 in, 5 out]
            n197 = property on="Use max power tracking" class="Bool (strict)"() -> ("Value"=w191:bool)  [unwired: 2 in, 2 out]
            n198 = case shown="True" w191 {
              frame False {
              }
              frame True {
                n199 = property on="Use Vmp from JV scan" class="Bool (strict)"("Value"=FALSE) -> ()  [unwired: 2 in, 2 out]
              }
            }
            n200 = property on="Use Vmp from JV scan" class="Bool (strict)"() -> ("Value"=w188:bool)  [unwired: 2 in, 2 out]
            n201 = property on="Use max power tracking" class="Bool (strict)"() -> ("Value"=w189:bool)  [unwired: 2 in, 2 out]
            n202 = Not Or(1:w189, 2:w188) -> (0:w190:bool)
            n203 = case shown="False" w190 {
              frame False {
                n204 = property on="Stabization voltage (V)" class="DigNum (strict)"("DisabledEnum"=T8."Disabled and Grayed Out" ("Disabled")) -> ()  [unwired: 2 in, 2 out]
              }
              frame True {
                n205 = property on="Stabization voltage (V)" class="DigNum (strict)"("DisabledEnum"=T8."Enabled" ("Disabled")) -> ()  [unwired: 2 in, 2 out]
              }
            }
          }
          event "Stop Scan 2": Value Change {
            n206 = event-data() -> ()  [unwired: 1 in, 5 out]
          }
        }
        n207 = property on="Stop Scan" class="Bool"("DisabledEnum"=T8."Disabled and Grayed Out" ("Disabled")) -> ()  [unwired: 2 in, 2 out]
      }
      frame "Measure" {
        w198 = T8."Disabled and Grayed Out" ("Disabled")
        # "Disable front panel objects during measurements\nto avoid possible crashes"
        # "\"Measure\" state"
        n208 = stacked-sequence {
          tunnel: [_ w240] -> w201
          tunnel: w200 -> [w203 _]
          tunnel: w197 -> [w202 _]
          frame #0 {
            # "Take measurements of elements in queue"
            n209 = local read "Queue"() -> (w204:T5)
            n210 = while {
              tunnel: w203 -> [w212]
              tunnel: w202 -> [w206]
              shift-right: [w207] -> _
              shift-left: w204 -> [w213]
              tunnel: w203 -> [w210]
              stop <- w209 stop-if-true
              # "Reset queue after every measurement"
              # "Build queue"
              n211 = call "Scans.vi"("Time zero (sec)"=w212, "Queue in"=w213) -> ("Queue out"=w211:T5)
              n212 = call "Sort queue by Time to next scan.vi"("Queue"=w211) -> ("Queue Out"=w208:T5)  [unwired: 4 in]
              n213 = Wait (ms)(milliseconds to wait=u32 1000) -> ()  [unwired: 1 out]
              n214 = local write "Queue"(w208) -> ()
              n215 = while {
                tunnel: w208 -> [w220] mode=indexing
                tunnel: w210 -> [w219]
                tunnel: ["Stop Scan"] -> w209
                shift-right: [w217] -> w207
                shift-left: w208 -> [w218]
                tunnel: w206 -> [w216]
                stop <- "Stop Scan" stop-if-true
                # "Loop through elements in queue until stop button is pressed"
                n216 = Wait (ms)(milliseconds to wait=u32 1000) -> ()  [unwired: 1 out]
                n217 = case shown="False" "Stop Scan" {
                  tunnel: w220 -> [w237 _]
                  tunnel: w219 -> [w232 _]
                  tunnel: w218 -> [w229 w238]
                  tunnel: [w221 w238] -> w217
                  tunnel: w216 -> [w228 _]
                  frame False {
                    # "Take measurements of all pixels\nfor given cell in queue"
                    # "Update queue"
                    n218 = Unbundle By Name(w237) -> ("User Name"=w227:string, "Cell Description"=w236:string, "Cell Position"=w235:i32, "Scan settings in queue"=w233:u16, "Sample Holder"=w234:dbl)
                    n219 = call "ReadServerErrorStatus.vi"() -> ("Error Status"=w224:string)  [unwired: 11 in]
                    n220 = call "ServerStatusMessage.vi"("Error Status"=w224) -> ("Message out"=→"Server Status:":string)  [unwired: 10 in]
                    n221 = control-ref of="Max. Power Stabilization"() -> (w225:refnum<vi>)
                    n222 = control-ref of="Table"() -> (w231:refnum<vi>)
                    n223 = control-ref of="J-V Curve"() -> (w226:refnum<vi>)
                    n224 = call "Measure all pixels on cell and save data.vi"("Cell details cluster in"=w237, "Username"=w227, "Cell Description"=w236, "JV Refnum"=w226, "Cell position"=w235, "Tbl Refnum"=w231, "Sample Holder"=w234, "Scan settings in queue"=w233, "Scan settings array"=w228, "Time Zero"=w232, "Jt Refnum"=w225) -> ("Cell details cluster out"=w230:T6)  [unwired: 2 in, 2 out]
                    n225 = call "Update queue information.vi"("Cell details cluster"=w230, "Queue"=w229) -> ("Queue Out"=w222:T5)  [unwired: 3 in]
                    n226 = call "Scans.vi"("Queue in"=w222) -> ("Queue out"=w221:T5)  [unwired: 1 in]
                  }
                  frame True {
                  }
                }
                n227 = local write "Queue"(w217) -> ()
              }
            }
          }
          frame #1 {
            w239 = T8."Enabled" ("Disabled")
            w240 = StateEnum."Idle"  # Enum
            n228 = property on="Cell Settings Array 1" class="Arr (strict)"("DisabledEnum"=w239) -> ()  [unwired: 2 in, 2 out]
            n229 = property on="Upload Spreadsheet path" class="Path"("DisabledEnum"=w239) -> ()  [unwired: 2 in, 2 out]
            n230 = property on="Upload from Spreadsheet?" class="Bool"("DisabledEnum"=w239) -> ()  [unwired: 2 in, 2 out]
            n231 = property on="Save Spreadsheet Path" class="Path"("DisabledEnum"=w239) -> ()  [unwired: 2 in, 2 out]
            n232 = property on="Save to Spreadsheet?" class="Bool"("DisabledEnum"=w239) -> ()  [unwired: 2 in, 2 out]
            n233 = property on="Cell Settings Array 2" class="Arr (strict)"("DisabledEnum"=w239) -> ()  [unwired: 2 in, 2 out]
            n234 = property on="Upload Spreadsheet path 2" class="Path"("DisabledEnum"=w239) -> ()  [unwired: 2 in, 2 out]
            n235 = property on="Upload from Spreadsheet? 2" class="Bool"("DisabledEnum"=w239) -> ()  [unwired: 2 in, 2 out]
            n236 = property on="Save Spreadsheet Path 2" class="Path"("DisabledEnum"=w239) -> ()  [unwired: 2 in, 2 out]
            n237 = property on="Save to Spreadsheet?  2" class="Bool"("DisabledEnum"=w239) -> ()  [unwired: 2 in, 2 out]
            n238 = property on="Cell Settings Array 3" class="Arr (strict)"("DisabledEnum"=w239) -> ()  [unwired: 2 in, 2 out]
            n239 = property on="Upload Spreadsheet path 3" class="Path"("DisabledEnum"=w239) -> ()  [unwired: 2 in, 2 out]
            n240 = property on="Upload from Spreadsheet? 3" class="Bool"("DisabledEnum"=w239) -> ()  [unwired: 2 in, 2 out]
            n241 = property on="Save Spreadsheet Path 3" class="Path"("DisabledEnum"=w239) -> ()  [unwired: 2 in, 2 out]
            n242 = property on="Save to Spreadsheet?  3" class="Bool"("DisabledEnum"=w239) -> ()  [unwired: 2 in, 2 out]
            n243 = property on="Cell Settings Array 4" class="Arr (strict)"("DisabledEnum"=w239) -> ()  [unwired: 2 in, 2 out]
            n244 = property on="Upload Spreadsheet path 4" class="Path"("DisabledEnum"=w239) -> ()  [unwired: 2 in, 2 out]
            n245 = property on="Upload from Spreadsheet? 4" class="Bool"("DisabledEnum"=w239) -> ()  [unwired: 2 in, 2 out]
            n246 = property on="Save Spreadsheet Path 4" class="Path"("DisabledEnum"=w239) -> ()  [unwired: 2 in, 2 out]
            n247 = property on="Save to Spreadsheet?  4" class="Bool"("DisabledEnum"=w239) -> ()  [unwired: 2 in, 2 out]
            n248 = property on="Start Scan" class="Bool"("DisabledEnum"=w239) -> ()  [unwired: 2 in, 2 out]
            n249 = property on="Stop Scan 2" class="Bool"("DisabledEnum"=w239) -> ()  [unwired: 2 in, 2 out]
            n250 = property on="Upload to the Queue" class="Bool (strict)"("DisabledEnum"=w239) -> ()  [unwired: 2 in, 2 out]
            n251 = property on="Scan Settings JV" class="Clust (strict)"("DisabledEnum"=w239) -> ()  [unwired: 2 in, 2 out]
            n252 = property on="Show saved settings" class="Ring (strict)"("DisabledEnum"=w239) -> ()  [unwired: 2 in, 2 out]
            n253 = property on="Save new settings" class="Bool"("DisabledEnum"=w239) -> ()  [unwired: 2 in, 2 out]
            n254 = property on="Save new settings as..." class="Str"("DisabledEnum"=w239) -> ()  [unwired: 2 in, 2 out]
          }
        }
        n255 = property on="Upload from Spreadsheet?" class="Bool"("DisabledEnum"=w198) -> ()  [unwired: 2 in, 2 out]
        n256 = property on="Save to Spreadsheet?" class="Bool"("DisabledEnum"=w198) -> ()  [unwired: 2 in, 2 out]
        n257 = property on="Cell Settings Array 1" class="Arr (strict)"("DisabledEnum"=w198) -> ()  [unwired: 2 in, 2 out]
        n258 = property on="Upload Spreadsheet path" class="Path"("DisabledEnum"=w198) -> ()  [unwired: 2 in, 2 out]
        n259 = property on="Save Spreadsheet Path" class="Path"("DisabledEnum"=w198) -> ()  [unwired: 2 in, 2 out]
        n260 = property on="Upload from Spreadsheet? 2" class="Bool"("DisabledEnum"=w198) -> ()  [unwired: 2 in, 2 out]
        n261 = property on="Save to Spreadsheet?  2" class="Bool"("DisabledEnum"=w198) -> ()  [unwired: 2 in, 2 out]
        n262 = property on="Upload Spreadsheet path 2" class="Path"("DisabledEnum"=w198) -> ()  [unwired: 2 in, 2 out]
        n263 = property on="Save Spreadsheet Path 2" class="Path"("DisabledEnum"=w198) -> ()  [unwired: 2 in, 2 out]
        n264 = property on="Cell Settings Array 2" class="Arr (strict)"("DisabledEnum"=w198) -> ()  [unwired: 2 in, 2 out]
        n265 = property on="Upload from Spreadsheet? 3" class="Bool"("DisabledEnum"=w198) -> ()  [unwired: 2 in, 2 out]
        n266 = property on="Save to Spreadsheet?  3" class="Bool"("DisabledEnum"=w198) -> ()  [unwired: 2 in, 2 out]
        n267 = property on="Upload Spreadsheet path 3" class="Path"("DisabledEnum"=w198) -> ()  [unwired: 2 in, 2 out]
        n268 = property on="Save Spreadsheet Path 3" class="Path"("DisabledEnum"=w198) -> ()  [unwired: 2 in, 2 out]
        n269 = property on="Cell Settings Array 3" class="Arr (strict)"("DisabledEnum"=w198) -> ()  [unwired: 2 in, 2 out]
        n270 = property on="Upload from Spreadsheet? 4" class="Bool"("DisabledEnum"=w198) -> ()  [unwired: 2 in, 2 out]
        n271 = property on="Save to Spreadsheet?  4" class="Bool"("DisabledEnum"=w198) -> ()  [unwired: 2 in, 2 out]
        n272 = property on="Upload Spreadsheet path 4" class="Path"("DisabledEnum"=w198) -> ()  [unwired: 2 in, 2 out]
        n273 = property on="Save Spreadsheet Path 4" class="Path"("DisabledEnum"=w198) -> ()  [unwired: 2 in, 2 out]
        n274 = property on="Cell Settings Array 4" class="Arr (strict)"("DisabledEnum"=w198) -> ()  [unwired: 2 in, 2 out]
        n275 = property on="Upload to the Queue" class="Bool (strict)"("DisabledEnum"=w198) -> ()  [unwired: 2 in, 2 out]
        n276 = property on="Start Scan" class="Bool"("DisabledEnum"=w198) -> ()  [unwired: 2 in, 2 out]
        n277 = property on="Stop Scan 2" class="Bool"("DisabledEnum"=w198) -> ()  [unwired: 2 in, 2 out]
        n278 = property on="Show saved settings" class="Ring (strict)"("DisabledEnum"=w198) -> ()  [unwired: 2 in, 2 out]
        n279 = property on="Save new settings as..." class="Str"("DisabledEnum"=w198) -> ()  [unwired: 2 in, 2 out]
        n280 = property on="Save new settings" class="Bool"("DisabledEnum"=w198) -> ()  [unwired: 2 in, 2 out]
      }
    }
  }
